vi "Check Error Response.vi"(8 "error in (no error)":errorcluster, 11 "read String":string) -> (0 "error out":errorcluster, 2 "Error Response":bool, 3 "String out":string)   [LabVIEW 2021, in "Environment Chamber.lvlib" / "Climatic Chamber.lvlib"]
uses:
  Climatic Chamber.lvlib
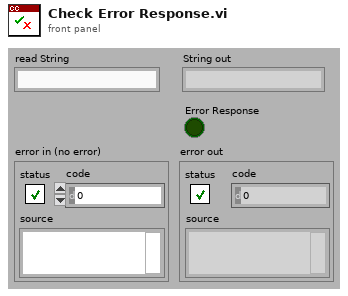
[diagram p1: front panel]
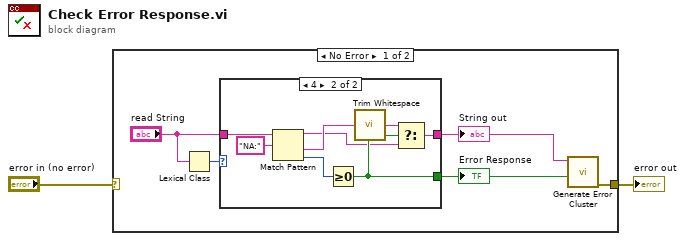
[diagram p0: block diagram]
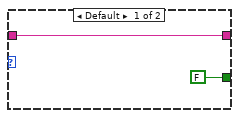
[diagram p2: hidden frame]
diagram:
  n1 = case shown="No Error" "error in (no error)" {
    selector: "error in (no error)" -> [_ w18]
    tunnel: [w3 w18] -> w2
    frame No Error {
      n2 = Lexical Class(1:"read String") -> (0:w7:i16)
      n3 = case shown="4" w7 {
        tunnel: [w9 w11] -> w4
        tunnel: "read String" -> [w9 w17]
        tunnel: [FALSE w14] -> w5
        frame Default {
        }
        frame 4 {
          n4 = Match Pattern(string=w17, regular expression="NA:") -> (before substring=w12:string, after substring=w13:string, offset past match=w15:i32)  [unwired: 1 in, 1 out]
          n5 = Greater Or Equal To 0?(x=w15) -> (x >= 0?=w14:bool)
          n6 = call <vilib>:"Trim Whitespace.vi"("string"=w13) -> ("trimmed string"=w10:string)  [unwired: 1 in]
          n7 = Select(t=w10, s=w14, f=w12) -> (s? t:f=w11:string)
        }
      }
      "String out" <- w4
      "Error Response" <- w5
      n8 = call "Generate Error Cluster.vi"("Error active?"=w5, "Error_message"=w4) -> ("error out"=w3:errorcluster)  [unwired: 9 in]
    }
    frame Error {
    }
  }
  "error out" <- w2
